vi "Find DAQ Devices.vi"(8 "Error In":errorcluster) -> (0 "Error Out":errorcluster, 2 "Stop?":bool, 3 "DAQmx Device Name":tag)   [LabVIEW 2017]
doc: "This VI returns information on all DAQ devices connected to the development computer. \n\nIf you do not wire any of the search inputs it will not return an element. It will, however, return the list of connected devices and serial numbers and a table of all the devices connected."
uses:
  <resource>/objmgr/daqmx.rc
panel:
  in  "OK Button":bool=TRUE
  in  "ConnectedDevices":u16(ring)
  out "All Device IDs":tag[](array[tag])
  # "Please select the correct connected device from the list:"
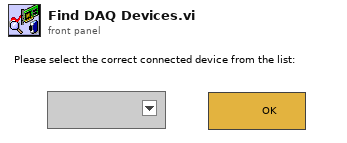
[diagram p1: front panel]
types:
  T1 = enum32{"Invalid", "Standard", "Closed", "Hidden", "Minimized", "Maximized"}
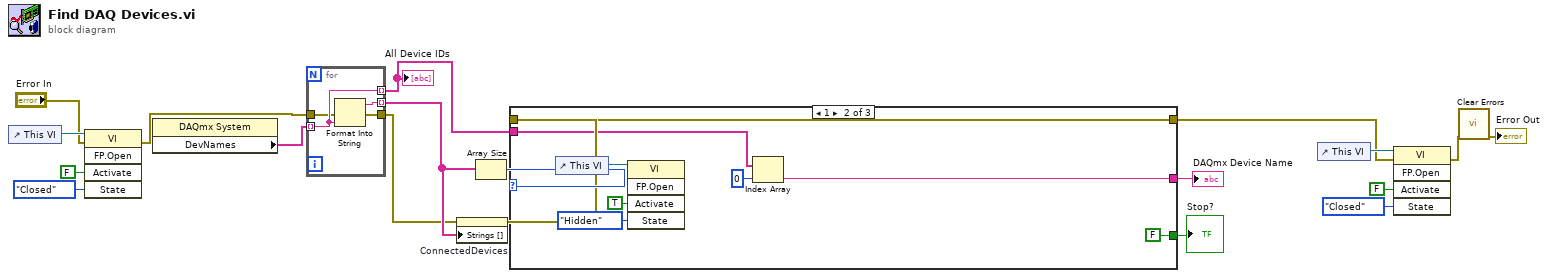
[diagram p0: block diagram]
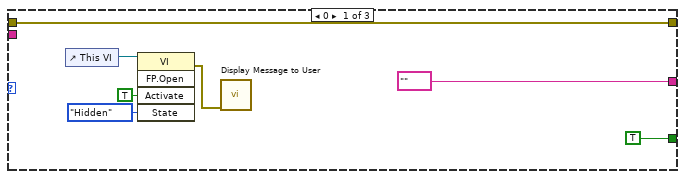
[diagram p2: hidden frame]
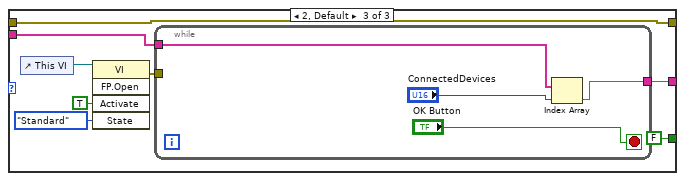
[diagram p3: hidden frame]
diagram:
  n1 = control-ref of="This VI"() -> (w7:refnum<vi>)
  n2 = invoke class="VI" method="FP.Open"(reference=w7, error in="Error In", "Activate"=FALSE ("Activate?"), "State"=T1."Closed") -> (error out=w5:errorcluster)  [unwired: 1 in, 4 out]
  n3 = property class="DAQmx System"() -> ("DevNames"=w19:tag[])  [unwired: 2 in, 2 out]
  n4 = for {
    tunnel: w19 -> [w22] mode=indexing
    tunnel: [w23] -> w18 mode=indexing
    tunnel: [w22] -> w16 mode=indexing
    tunnel: w5 -> [w21]
    tunnel: [w20] -> w4
    n5 = Format Into String(error in=w21, w22) -> (resulting string=w23:string, error out=w20:errorcluster)  [unwired: 2 in]
  }
  "All Device IDs" <- w16
  n6 = property on="ConnectedDevices" class="Ring (strict)"(error in=w4, "Strings []"=w18) -> (error out=w3:errorcluster)  [unwired: 1 in, 1 out]
  n7 = Array Size(array=w18) -> (size(s)=w17:i32)
  n8 = case shown="1" w17 {
    tunnel: w16 -> [_ w38 w45]
    tunnel: [tag "" w36 w44] -> w15
    tunnel: w3 -> [w29 w35 w46]
    tunnel: [w29 w35 w46] -> w11
    tunnel: [TRUE FALSE FALSE] -> w1
    frame 0 {
      n9 = control-ref of="This VI"() -> (w27:refnum<vi>)
      n10 = invoke class="VI" method="FP.Open"(reference=w27, "Activate"=TRUE ("Activate?"), "State"=T1."Hidden") -> (error out=w24:errorcluster)  [unwired: 2 in, 4 out]
      n11 = call "Display Message to User"("error in (no error)"=w24) -> ()  [unwired: 9 in, 2 out]
    }
    frame 1 {
      n12 = control-ref of="This VI"() -> (w33:refnum<vi>)
      n13 = invoke class="VI" method="FP.Open"(reference=w33, "Activate"=TRUE ("Activate?"), "State"=T1."Hidden") -> ()  [unwired: 2 in, 5 out]
      n14 = Index Array(array=w38, index=0) -> (element=w36:tag)
    }
    frame 2, Default {
      n15 = control-ref of="This VI"() -> (w41:refnum<vi>)
      n16 = invoke class="VI" method="FP.Open"(reference=w41, "Activate"=TRUE ("Activate?"), "State"=T1."Standard") -> (error out=w40:errorcluster)  [unwired: 2 in, 4 out]
      n17 = while {
        tunnel: w45 -> [w49]
        tunnel: [w48] -> w44
        tunnel: w40 -> [_]
        stop <- "OK Button" stop-if-true
        n18 = Index Array(array=w49, index="ConnectedDevices") -> (element=w48:tag)
      }
    }
  }
  "DAQmx Device Name" <- w15
  "Stop?" <- w1
  n19 = control-ref of="This VI"() -> (w12:refnum<vi>)
  n20 = invoke class="VI" method="FP.Open"(reference=w12, error in=w11, "Activate"=FALSE ("Activate?"), "State"=T1."Closed") -> (error out=w10:errorcluster)  [unwired: 1 in, 4 out]
  n21 = call <vilib>:"Clear Errors.vi"("error in (no error)"=w10) -> ("error out"=→"Error Out":errorcluster)  [unwired: 5 in, 1 out]
